vi "Read Time.vi"(8 "error in (no error)":errorcluster, 11 "ControlKeyDownMsg in":refnum<class "VIKeyDownMsg.lvclass">) -> (0 "error out":errorcluster, 2 "Time":u32, 3 "ControlKeyDownMsg out":refnum<class "VIKeyDownMsg.lvclass">)   [LabVIEW 2020, in "ActorEvents.lvlib" / "VIKeyDownMsg.lvclass"]
uses:
  VIKeyDownMsg.lvclass
  VIKeyDownMsg.lvclass/VIKeyDownMsg.ctl
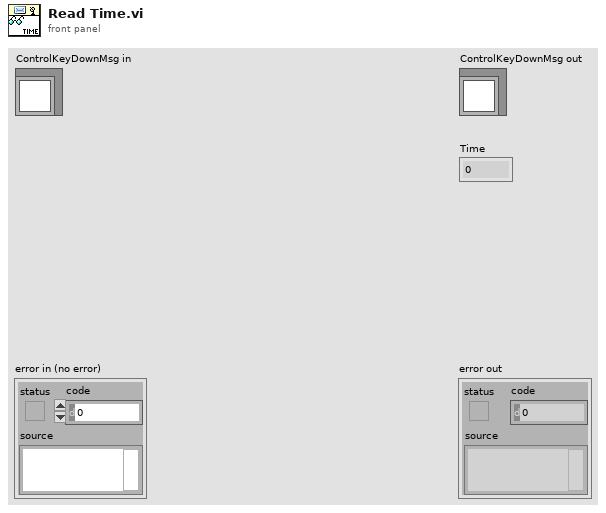
[diagram p1: front panel]
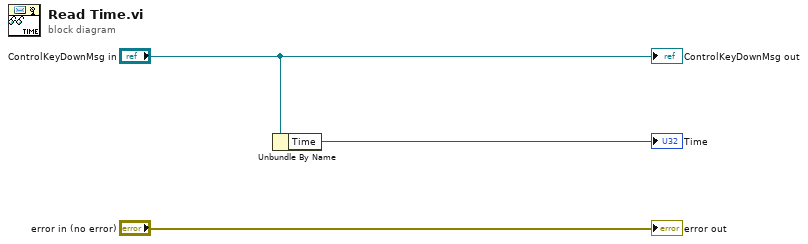
[diagram p0: block diagram]
diagram:
  n1 = Unbundle By Name("ControlKeyDownMsg in") -> ("Time"=→"Time":u32)
  "error out" <- "error in (no error)"
  "ControlKeyDownMsg out" <- "ControlKeyDownMsg in"
